vi "Write.vi"(6 "Append Index":i32, 8 "error in (no error)":errorcluster, 9 "Notes":string, 10 "Data (Dictionary)":T1[](array[typedef]), 11 "Data.TDMS in":refnum<class "Data.PG.lvclass">) -> (0 "error out":errorcluster, 3 "Data.TDMS out":refnum<class "Data.PG.lvclass">, 5 "Path out":path)   [LabVIEW 2020, in "Data.PG.lvclass"]
uses:
  Data.PG.lvclass
  C:/user/patrick/git/LV-to-ITX/src/Data/Data.lvclass
  Data/Typedefs/Dictionary--cluster.ctl
  <vilib>/JDP Science/PostgreSQL Library/Connection/PQ Connection.lvclass
  Data.PG.lvclass/Data.PG.ctl
  Data/Typedefs/Operation--enum.ctl
  Data/Data.lvclass/Data.ctl
  <vilib>/JDP Science/PostgreSQL Library/Result/PQ Result.lvclass/PQ Result.ctl
  <vilib>/JDP Science/PostgreSQL Library/Connection/Execute Command (No results).vi
  <vilib>/JDP Science/PostgreSQL Library/Result/Clear.vi
  <vilib>/JDP Science/PostgreSQL Library/Connection/Execute Command (Result).vi
  <vilib>/JDP Science/PostgreSQL Library/Connection/Execute (no results).vi
  <vilib>/JDP Science/PostgreSQL Library/Connection/Execute (Return first result with rows).vi
  <vilib>/JDP Science/PostgreSQL Library/Connection/Single Command with parameters.vi
  Data/Data.lvclass
panel:
  in  "Table name":string="my_table"
  out "INSERTS/sec":dbl format="%#_3p"
  out "Time per INSERT":dbl format="%#_3p"
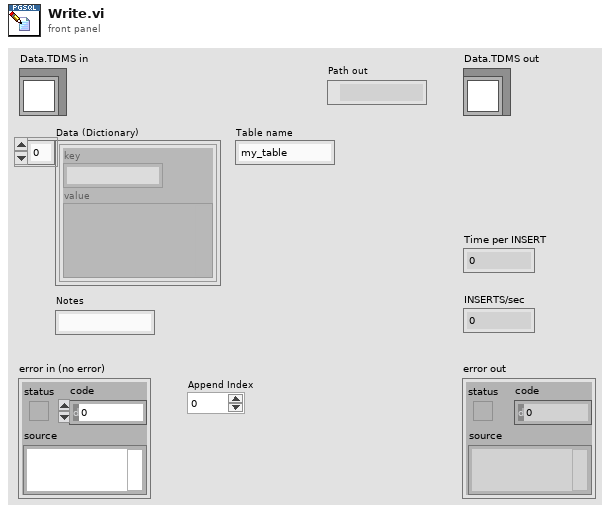
[diagram p1: front panel]
types:
  T1 = typedef "Data.lvclass/Dictionary--cluster.ctl" = cluster{"key":string, "value":variant}
  T2 = typedef "Data.lvclass/Operation--enum.ctl" = enum16{"Read", "Write", "Write + Append"}
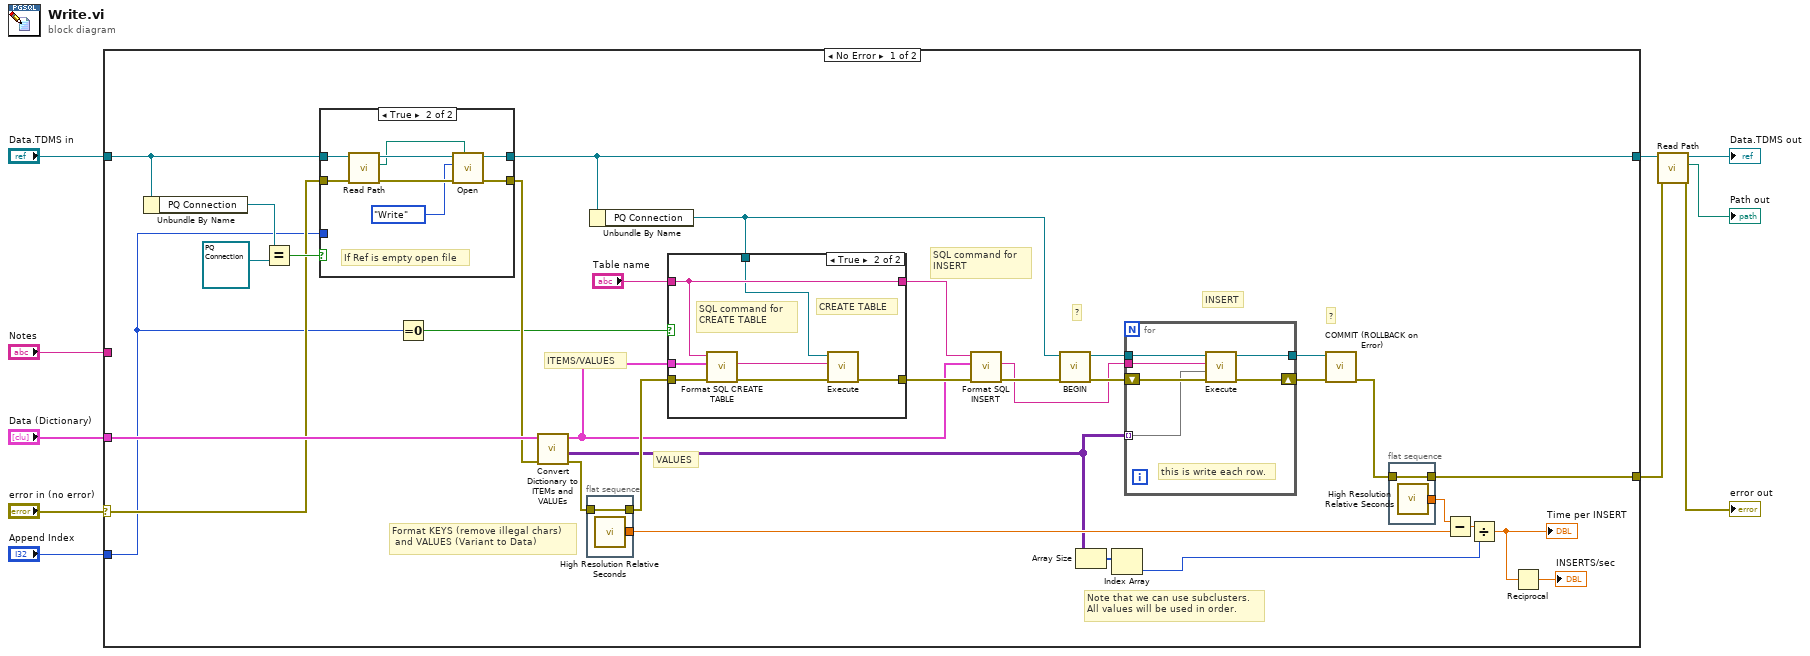
[diagram p0: block diagram]
diagram:
  n1 = case shown="No Error" "error in (no error)" {
    selector: "error in (no error)" -> [w27 w74]
    tunnel: [w33 w74] -> w1
    tunnel: "Data.TDMS in" -> [w29 w73]
    tunnel: [w24 w73] -> w6
    tunnel: "Data (Dictionary)" -> [w43 _]
    tunnel: "Notes" -> [_ _]
    tunnel: "Append Index" -> [w13 _]
    frame No Error {
      # "SQL command for\nINSERT"
      # "?"
      # "?"
      # "INSERT"
      # "Format KEYS (remove illegal chars)\n and VALUES (Variant to Data)"
      # "VALUES"
      # "ITEMS/VALUES"
      # "Note that we can use subclusters.\nAll values will be used in order."
      n2 = Unbundle By Name(w29) -> ("PQ Connection"=w30:refnum<class "PQ Connection.lvclass">)
      n3 = Equal?(x=w30, y=refnum<class "PQ Connection.lvclass"> refnum ("PQ Connection")) -> (x = y?=w31:bool)
      n4 = case shown="True" w31 {
        tunnel: w29 -> [w57 w66]
        tunnel: [w57 w59] -> w24
        tunnel: [w58 w63] -> w42
        tunnel: w27 -> [w58 w62]
        tunnel: w13 -> [_ _]
        frame False {
        }
        frame True {
          # "If Ref is empty open file"
          n5 = call "Read Path.vi"("error in (no error)"=w62, "Data Save"=w66) -> ("error out"=w65:errorcluster, "Path"=w61:path, "Data Save out"=w64:refnum<class "Data.PG.lvclass">)  [unwired: 7 in]
          n6 = call-dynamic "Open.vi"("Path"=w61, "error in (no error)"=w65, "Operation"=Operation--enum."Write", "Data.TDMS in"=w64) -> ("error out"=w63:errorcluster, "Data.TDMS out"=w59:refnum<class "Data.PG.lvclass">)  [unwired: 6 in]
        }
      }
      n7 = Equal To 0?(x=w13) -> (x = 0?=w12:bool)
      n8 = call "Convert Dictionary to ITEMs and VALUEs.vi"("error in (no error)"=w42, "Data (Dictionary)"=w43) -> ("error out"=w41:errorcluster, "2D Array of Variants"=w14:variant[][], "Data (Dictionary)"=w15:T1[])  [unwired: 6 in, 1 out]
      n9 = flat-sequence {
        tunnel: w41 -> [w55]
        tunnel: [w56] -> w36
        tunnel: [w55] -> w28
        frame #0 {
          n10 = call <vilib>:"High Resolution Relative Seconds.vi"() -> ("relative seconds"=w56:dbl)
        }
      }
      n11 = Unbundle By Name(w24) -> ("PQ Connection"=w16:refnum<class "PQ Connection.lvclass">)
      n12 = case shown="True" w12 {
        tunnel: w28 -> [w45 w52]
        tunnel: [w45 w49] -> w26
        tunnel: "Table name" -> [w44 w47]
        tunnel: w16 -> [_ w46]
        tunnel: w15 -> [_ w48]
        tunnel: [w44 w47] -> w11
        frame False {
        }
        frame True {
          # "SQL command for\nCREATE TABLE"
          # "CREATE TABLE"
          n13 = call "Format SQL CREATE TABLE.vi"("error in (no error)"=w52, "Data (Dictionary)"=w48, "Table name"=w47) -> ("error out"=w51:errorcluster, "SQL"=w50:string)  [unwired: 7 in]
          n14 = call-poly <vilib>:"Execute.vi"("error in (no error)"=w51, "SQL"=w50, "PQ Connection in"=w46) -> ("error out"=w49:errorcluster)  [unwired: 7 in, 1 out]
        }
      }
      n15 = call "Format SQL INSERT.vi"("error in (no error)"=w26, "Data (Dictionary)"=w15, "table name"=w11) -> ("error out"=w25:errorcluster, "SQL"=w21:string)  [unwired: 7 in]
      n16 = call <vilib>:"BEGIN.vi"("error in (no error)"=w25, "PQ Connection in"=w16) -> ("error out"=w38:errorcluster, "PQ Connection out"=w23:refnum<class "PQ Connection.lvclass">)  [unwired: 8 in]
      n17 = Array Size(array=w14) -> (size(s)=w19:i32[])
      n18 = Index Array(array=w19) -> (element=w17:i32)  [unwired: 1 in]
      n19 = for {
        tunnel: w21 -> [w71]
        shift-right: [w68] -> w34
        shift-left: w38 -> [w69]
        tunnel: w23 -> [w70]
        tunnel: [w72] -> w22
        tunnel: w14 -> [w67] mode=indexing
        # "this is write each row."
        n20 = call-poly <vilib>:"Execute.vi"("error in (no error)"=w69, "Parameters"=w67, "SQL"=w71, "PQ Connection in"=w70) -> ("error out"=w68:errorcluster, "PQ Connection out"=w72:refnum<class "PQ Connection.lvclass">)  [unwired: 6 in]
      }
      n21 = call <vilib>:"COMMIT (ROLLBACK on Error).vi"("error in (no error)"=w34, "PQ Connection in"=w22) -> ("error out"=w18:errorcluster)  [unwired: 8 in, 1 out]
      n22 = flat-sequence {
        tunnel: w18 -> [w54]
        tunnel: [w54] -> w33
        tunnel: [w53] -> w35
        frame #0 {
          n23 = call <vilib>:"High Resolution Relative Seconds.vi"() -> ("relative seconds"=w53:dbl)
        }
      }
      n24 = Subtract(x=w35, y=w36) -> (x-y=w37:dbl)
      n25 = Divide(x=w37, y=w17) -> (x/y=w39:dbl)
      "Time per INSERT" <- w39
      n26 = Reciprocal(x=w39) -> (1/x=→"INSERTS/sec":dbl)
    }
    frame Error {
    }
  }
  n27 = call "Read Path.vi"("error in (no error)"=w1, "Data Save"=w6) -> ("error out"=→"error out":errorcluster, "Path"=→"Path out":path, "Data Save out"=→"Data.TDMS out":refnum<class "Data.PG.lvclass">)  [unwired: 7 in]
